vi "StreamEngine.CreateQueue.vi"(8 "error in (no error)":errorcluster) -> (0 "error out":errorcluster, 3 "Q Refs":T1)   [LabVIEW 2025, in "XNET Bus Monitor Client.lvlib"]
uses:
  XNET Bus Monitor Client.lvlib
  Types/StreamEngine.CmdQueueData.ctl
  Types/StreamEngine.CmdQueueData.Cmd.ctl
  Types/StreamEngine.QueueRefs.ctl
  Types/SubProcessEngine.CmdQueueData.ctl
  Types/SubProcessEngine.CmdQueueData.Cmd.ctl
  Types/SubProcessEngine.QueueRefs.ctl
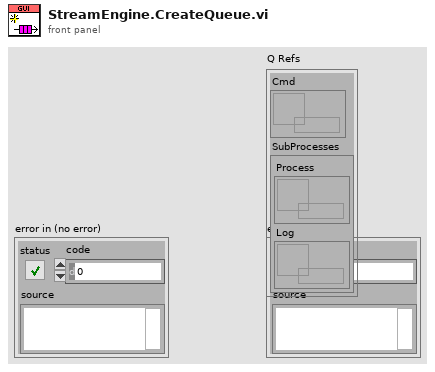
[diagram p1: front panel]
types:
  T1 = typedef "XNET Bus Monitor Client.lvlib/StreamEngine.QueueRefs.ctl" = cluster{"Cmd":refnum<queue>, "SubProcesses":T2}
  T2 = typedef "XNET Bus Monitor Client.lvlib/SubProcessEngine.QueueRefs.ctl" = cluster{"Process":refnum<queue>, "Log":refnum<queue>}
  T3 = typedef "XNET Bus Monitor Client.lvlib/SubProcessEngine.CmdQueueData.ctl" = cluster{"Cmd":T4, "Parameters":variant}
  T4 = typedef "XNET Bus Monitor Client.lvlib/SubProcessEngine.CmdQueueData.Cmd.ctl" = enum16{"Arm", "Publish", "Stop", "Exit"}
  T5 = typedef "XNET Bus Monitor Client.lvlib/StreamEngine.CmdQueueData.ctl" = cluster{"Cmd":T6, "Parameters":variant}
  T6 = typedef "XNET Bus Monitor Client.lvlib/StreamEngine.CmdQueueData.Cmd.ctl" = enum8{"Start Stream", "Stop Stream", "Exit"}
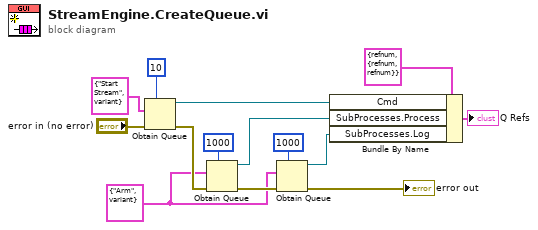
[diagram p0: block diagram]
diagram:
  w1 = T3 {"Cmd"=enum."Arm", "Parameters"=variant(cluster{"can_comm_state":cluster{"fault_code":i32, "fault":bool, "comm_state":enum32{"Error_Active", "Error_Passive", "Bus_Off", "Init"}, "last_comm_error":enum32{"None", "Stuff", "Form", "ACK", "Bit1", "Bit0", "CRC"}, "receive_error_counter":u32, "transmit_error_counter":u32, "transceiver_error":bool, "sleep":bool}, "frame":cluster{"timestamp":dbl, "payload":u8[], "identifier":u32, "frame_type":u32, "extended":bool, "echo":bool}[], "error":errorcluster} {"can_comm_state"={"fault_code"=0, "fault"=FALSE, "comm_state"=enum."Error_Active", "last_comm_error"=enum."None", "receive_error_counter"=0, "transmit_error_counter"=0, "transceiver_error"=FALSE, "sleep"=FALSE}, "frame"=[], "error"={"status"=FALSE, "code"=0, "source"=""}})}
  n1 = Obtain Queue(max queue size (-1, unlimited)=10, element data type=T5 {"Cmd"=enum."Start Stream", "Parameters"=variant}, error in (no error)="error in (no error)") -> (queue out=w8:refnum<queue>, error out=w12:errorcluster)  [unwired: 2 in, 1 out]
  n2 = Obtain Queue(max queue size (-1, unlimited)=1000, element data type=w1, error in (no error)=w12) -> (queue out=w7:refnum<queue>, error out=w5:errorcluster)  [unwired: 2 in, 1 out]
  n3 = Obtain Queue(max queue size (-1, unlimited)=1000, element data type=w1, error in (no error)=w5) -> (queue out=w3:refnum<queue>, error out=→"error out":errorcluster)  [unwired: 2 in, 1 out]
  n4 = Bundle By Name(cluster=T1 {"Cmd"=refnum, "SubProcesses"={"Process"=refnum, "Log"=refnum}} ("Q Refs"), "Cmd"=w8, "SubProcesses.Process"=w7, "SubProcesses.Log"=w3) -> (→"Q Refs":T1)
